vi "Add FPGA Configuration.vi"(8 "error in (no error)":errorcluster, 10 "FPGA Configuration in":refnum<k24>, 11 "Item Ref in":T1 format="%.0x") -> (0 "error out":errorcluster, 2 "FPGA Configuration out":refnum<k24>, 3 "Item Ref out":T1 format="%.0x")   [LabVIEW 2014, in "SLSC configuration System Explorer.lvlib"]
uses:
  SLSC configuration System Explorer.lvlib
  <vilib>/NI Veristand/Custom Device API/Custom Device Item Ref.ctl
  <vilib>/NI Veristand/Custom Device API/Custom Device API.lvlib
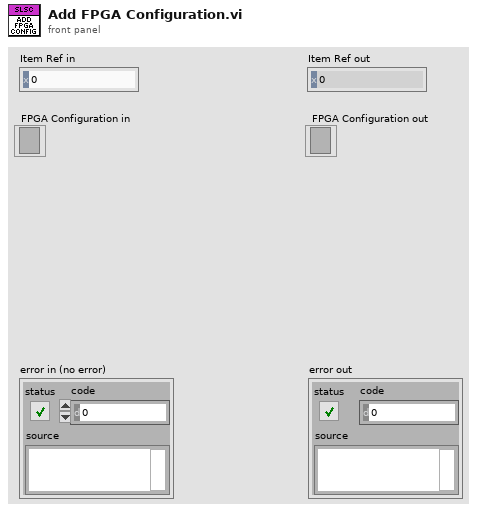
[diagram p1: front panel]
types:
  T1 = typedef "Custom Device API.lvlib/Custom Device Item Ref.ctl" = u64
  T2 = typedef "SLSC configuration System Explorer.lvlib/SLSC Bitfile Info.ctl" = cluster{"FPGA Settings":string, "FIFO Name":string, "Max # of Racks":u8, "UEGO Simulation Names":string[]}
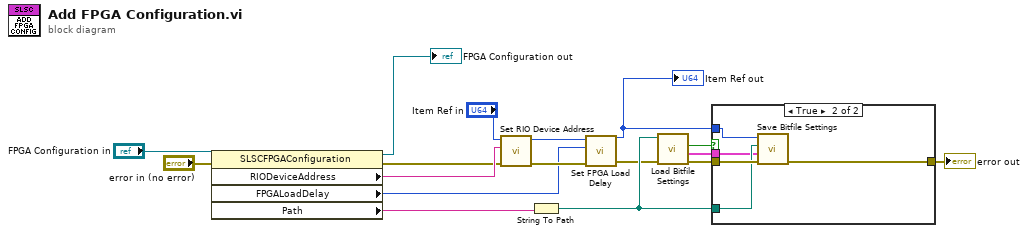
[diagram p0: block diagram]
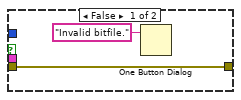
[diagram p2: hidden frame]
diagram:
  n1 = property class="SLSCFPGAConfiguration"(reference="FPGA Configuration in", error in="error in (no error)") -> (reference out=→"FPGA Configuration out":refnum<k24>, error out=w6:errorcluster, "RIODeviceAddress"=w7:string, "FPGALoadDelay"=w8:u16, "Path"=w10:string)
  n2 = call "Set RIO Device Address.vi"("error in (no error)"=w6, "RIO Device Address"=w7, "Item Ref in"="Item Ref in") -> ("error out"=w9:errorcluster, "Item Ref out"=w12:T1)  [unwired: 7 in]
  n3 = String To Path(string=w10) -> (path=w16:path)
  n4 = call "Set FPGA Load Delay.vi"("error in (no error)"=w9, "FPGA Load Delay (s)"=w8, "Item Ref in"=w12) -> ("error out"=w11:errorcluster, "Item Ref out"=w15:T1)  [unwired: 7 in]
  "Item Ref out" <- w15
  n5 = call "Load Bitfile Settings.vi"("error in (no error)"=w11, "bitfile path"=w16) -> ("error out"=w14:errorcluster, "Bitfile Info"=w17:T2, "Valid?"=w13:bool)  [unwired: 6 in, 1 out]
  n6 = case shown="True" w13 {
    tunnel: w14 -> [w18 w24]
    tunnel: w15 -> [_ w23]
    tunnel: w16 -> [_ w22]
    tunnel: w17 -> [_ w21]
    tunnel: [w18 w20] -> w1
    frame False {
      n7 = One Button Dialog(message="Invalid bitfile.") -> ()  [unwired: 1 in, 1 out]
    }
    frame True {
      n8 = call "Save Bitfile Settings.vi"("error in (no error)"=w24, "Bitfile Info"=w21, "Path"=w22, "Device Ref in"=w23) -> ("error out"=w20:errorcluster)  [unwired: 6 in, 1 out]
    }
  }
  "error out" <- w1
